vi "PDF_Interface_PDF Protokoll EPA1065_InterferenceVerification.vi"(8 "error in (no error)":errorcluster caption="Fehler (Eingang, kein Fehler)", 10 "Signalverlaufsdiagramm (Eingang)":refnum<vi>, 11 "Save PDF File Path":path) -> (0 "error out":errorcluster caption="Fehler (Ausgang)")   [LabVIEW 2020, in "EPA 1065.lvlib" / "HovaCAL Interference verificaton.lvlib"]
uses:
  HovaCAL Interference verificaton.lvlib
  Tabelle.ctl
  Tabelle Referenz.ctl
  Sprachverwaltung/FGV Aktion Tabelle zerlegen.ctl
  Aktion Index uebersetzten.ctl
  Aktion FGV Interference.ctl
  PDF_Interface/PDF Protokoll Standard Kopf Optionen.ctl
  <vilib>/Simplicity AI/SAI_PDF_API/Classes/Context/Controls/SAI_PDF_PDF Details.ctl
  PDF_Interface/PDF Interface Helper/PDFContentType.ctl
  PDF_Interface/PDF Interface Helper/PDFTableContentType.ctl
  PDF_Interface/PDF Interface Helper/PDFResults.ctl
  PDF_Interface/PDF Interface Helper/PDFResultPictures.ctl
  PDF_Interface/PDF Interface Helper/PDFCommentPosition.ctl
  PDF_Interface/PDF Interface Helper/PDFPageBreak.ctl
  PDF_Interface/PDF Interface Helper/PDFTablePictures.ctl
  PDF_Interface/PDF Interface Helper/PDFBemerkung.ctl
  <vilib>/Simplicity AI/SAI_PDF_API/Classes/Context/Controls/SAI_PDF_Text Align.ctl
  <vilib>/Simplicity AI/SAI_PDF_API/Classes/Context/Controls/SAI_PDF_Font.ctl
  <vilib>/Simplicity AI/SAI_PDF_API/Classes/Context/Controls/SAI_PDF_Font Encoding.ctl
  PDF_Interface/PDF Interface Helper/PDFGraph.ctl
  Sprachverwaltung/Sprachverwaltung.lvlib
  PDF_Interface/PDF Interface.lvlib
  PDF_Interface/PDF Interface Helper/PDF Interface Helper.lvlib
  <vilib>/Simplicity AI/SAI_PDF_API/Classes/Context/Context.lvclass
  Linearisierung V2/Protokoll/Protokoll.lvlib
panel:
  out "Kontroll Interferent":T1 caption="Kontroll-Interferent"
  out "Referenz Interferent":T2 caption="Referenz-Interferent"
  out "Komponente":T1
  out "Header Tabelle":string[][](table) caption="Tabelle"
  # "HovaCAL Interference Verification"
  # "Result"
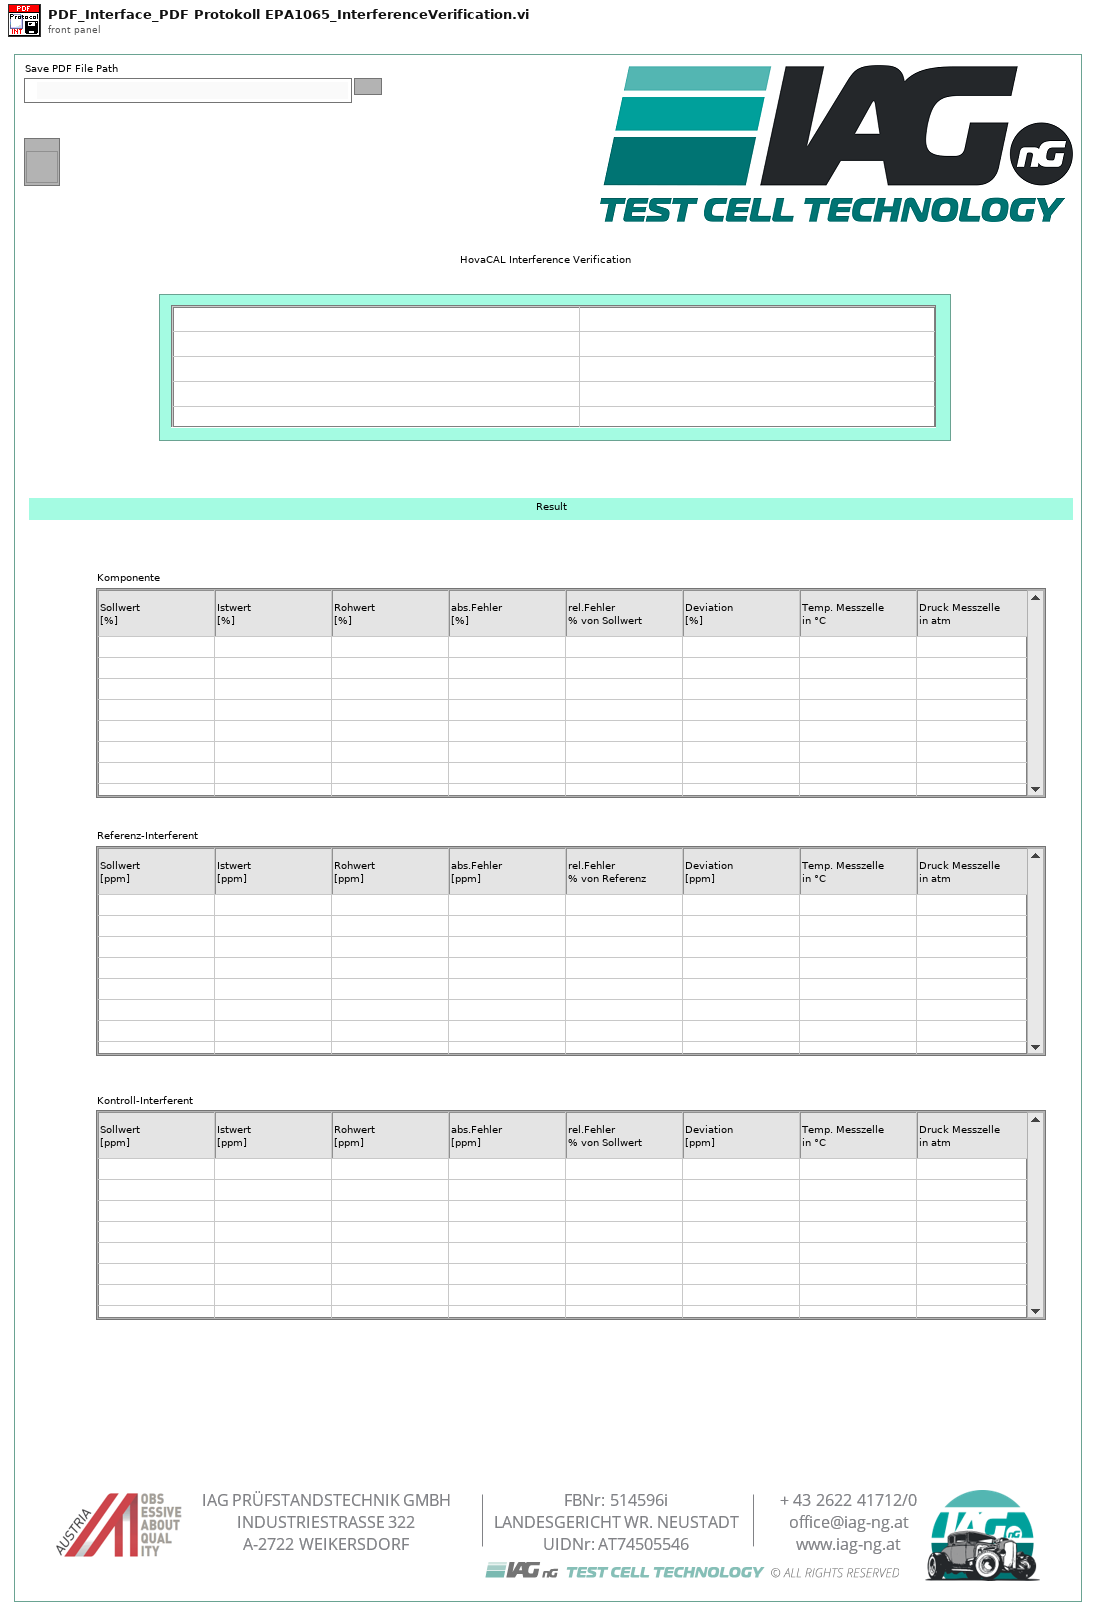
[diagram p1: front panel]
types:
  T1 = typedef "EPA 1065.lvlib/HovaCAL Interference verificaton.lvlib/Tabelle.ctl" = string[][]
  T2 = typedef "EPA 1065.lvlib/HovaCAL Interference verificaton.lvlib/Tabelle Referenz.ctl" = string[][]
  T3 = typedef "EPA 1065.lvlib/HovaCAL Interference verificaton.lvlib/Aktion FGV Interference.ctl" = enum16{"Lesen", "TestKonfig", "TestSetting", "Einheiten", "Ergebnis", "Laden", "Tabelle", "Speichern", "löschen"}
  T4 = typedef "EPA 1065.lvlib/HovaCAL Interference verificaton.lvlib/Aktion Index uebersetzten.ctl" = enum16{"lesen", "schreiben", "auswerten", "Referenzwert", "KompIndex", "RefInterferIndex", "KontrInterfIndex"}
  T5 = typedef "Sprachverwaltung.lvlib/FGV Aktion Tabelle zerlegen.ctl" = enum16{"laden", "vereinzeln", "speichern"}
  T6 = typedef "EPA 1065.lvlib/HovaCAL Interference verificaton.lvlib/Komponenten.ctl" = cluster{"Komponente":T7, "Komponente Index":i32, "Referenz Interferent":T7, "Refernz Interferent Index":i32, "Kontroll Interferent":T7, "Kontroll Interferent Index":i32, "Einheit Komponente":string, "Einheit Refernz Interferrent":string, "Einheit Kontroll Interferrent":string}
  T7 = typedef "String - Ausgabefeld.ctl" = string
  T8 = typedef "EPA 1065.lvlib/HovaCAL Interference verificaton.lvlib/TestSetting.ctl" = cluster{"Bearbeiter:":string, "Pfad:":path, "Textname:":string, "Analysator":T9}
  T9 = typedef "System Einstellungen V2.lvlib/Analysatoren.ctl" = string
  T10 = typedef "EPA 1065.lvlib/HovaCAL Interference verificaton.lvlib/TestKonfig.ctl" = cluster{"TestKonfig H2O":T11, "TestKonfig Interferent":T17}
  T11 = typedef "EPA 1065.lvlib/HovaCAL Interference verificaton.lvlib/TestKonfig H2O.ctl" = cluster{"Modus":T12, "Komponente:":u16, "Eingangs Konzentration:":dbl, "Einheit":T13, "Anzahl Stufen":sgl, "Zeitdauer Stufen":sgl, "Max Fehler":sgl, "zusätzliche Zeitdauer Erster Punkt":sgl, "Punkte umkehren":bool, "Stufen Tabelle":T14, "HovaCAL Flow Input Cluster":T15, "HovaCAL Temperature":T16}
  T12 = typedef "EPA 1065.lvlib/HovaCAL Interference verificaton.lvlib/Modus.ctl" = u16
  T13 = typedef "Linearisierung v2.lvlib/SpanEinstellungen.lvlib/Einheit.ctl" = enum16{"ppm", "%"}
  T14 = typedef "Linearisierung v2.lvlib/Gasteiler.lvlib/Stufen Tabelle 10 Stufen.ctl" = string[][]
  T15 = typedef "Linearisierung v2.lvlib/Gasteiler.lvlib/HovaCAL_Interface.lvlib/Controls.lvlib/Flow Einstellung.ctl" = cluster{"HovaCAL Flow Input Cluster":dbl}
  T16 = typedef "Linearisierung v2.lvlib/Gasteiler.lvlib/HovaCAL_Interface.lvlib/Controls.lvlib/Temp Sollwerte Anzeige.ctl" = dbl[]
  T17 = typedef "EPA 1065.lvlib/HovaCAL Interference verificaton.lvlib/TestKonfig Interferents.ctl" = cluster{"MFC1":enum16{"MFC 1"}, "Eingangs Konzentration MFC1":dbl, "Einheit MFC1 Eingang":T13, "Ausgangs Konzentration MFC1":dbl, "Einheit MFC1 Ausgang":T13, "MFC2":T18, "Referenz-Interferent:":u16, "Gasflaschen Nr MFC2":string, "Accuracy MFC2":string, "Eingangs Konzentration MFC2":dbl, "Einheit MFC2 Eingang":T13, "Ausgangs Konzentration MFC2":dbl, "Einheit MFC2 Ausgang":T13, "MFC3":T18, "Kontroll-Interferent:":u16, "Gasflaschen Nr MFC3":string, "Accuracy MFC3":string, "Eingangs Konzentration MFC3":dbl, "Einheit MFC3 Eingang":T13, "Ausgangs Konzentration MFC3":dbl, "Einheit MFC3 Ausgang":T13, "Gasflasche MFC2":T19, "Gasflasche MFC3":T19}
  T18 = typedef "EPA 1065.lvlib/HovaCAL Interference verificaton.lvlib/MFCAuswahl.ctl" = u16
  T19 = typedef "System Einstellungen V2.lvlib/Gasflasche Auswahl.ctl" = u16
  T20 = typedef "PDF Interface.lvlib/PDF Protokoll Standard Kopf Optionen.ctl" = cluster{"Analysator":bool, "FT-IR Rezept":bool, "Gasteiler":bool, "Gas Komponente":bool, "Gas Flasche":bool, "LIN Protokoll":bool, "Operator":bool}
  T21 = typedef "PDF Interface.lvlib/PDF Interface Helper.lvlib/PDFPageBreak.ctl" = enum16{"none", "before", "after", "after comment"}
  T22 = typedef "PDF Interface.lvlib/PDF Interface Helper.lvlib/PDFCommentPosition.ctl" = enum16{"before", "after"}
  T23 = typedef "PDF Interface.lvlib/PDF Interface Helper.lvlib/PDFGraph.ctl" = cluster{"GraphCtl Refnum":refnum<vi>, "Wrap Text (F:No)":bool, "Hide Grid (F:No)":bool, "Scale (100%)":sgl, "Align (Left)":T24, "PositionBemerkung":T22, "PageBreak":T21}
  T24 = typedef "SAI_PDF_Toolkit.lvlib/Context.lvclass/SAI_PDF_Text Align.ctl" = i32
  T25 = typedef "PDF Interface.lvlib/PDF Interface Helper.lvlib/PDFContentType.ctl" = cluster{"Titel":string, "Header Table":string[][], "Table Array":T26[], "Bemerkungen":T30[]}
  T26 = typedef "PDF Interface.lvlib/PDF Interface Helper.lvlib/PDFTableContentType.ctl" = cluster{"TableHeader":string[], "Table":string[][], "Relative Column Widths (%)":sgl[], "Results":T27, "PositionBemerkung":T22, "PageBreak":T21, "TablePictures":T29, "Horizontal Align":i32}
  T27 = typedef "PDF Interface.lvlib/PDF Interface Helper.lvlib/PDFResults.ctl" = cluster{"Results":cluster{"Result Text":string, "Result":bool}[], "ResultPictures":T28, "use Pictures":bool, "Image Scale (%)":sgl, "Autoscale? (T)":bool, "Horizontal Align":i32, "Position":i32}
  T28 = typedef "PDF Interface.lvlib/PDF Interface Helper.lvlib/PDFResultPictures.ctl" = cluster{"Yes Ctl Refnum":refnum<vi>, "No Ctl Refnum":refnum<vi>}
  T29 = typedef "PDF Interface.lvlib/PDF Interface Helper.lvlib/PDFTablePictures.ctl" = cluster{"Ctl Refnum In":refnum<vi>[], "RowOrColumn":enum16{"Row", "Column"}, "IndexToInsert":u16, "Image Scale (%)":sgl[], "Autoscale? (T)":bool[], "Horizontal Align":i32}
  T30 = typedef "PDF Interface.lvlib/PDF Interface Helper.lvlib/PDFBemerkung.ctl" = cluster{"Bemerkung Text":string, "Align (Left)":T24, "Add Line Feeds (F:No)":bool, "Font":T31}
  T31 = typedef "SAI_PDF_Toolkit.lvlib/Context.lvclass/SAI_PDF_Font.ctl" = cluster{"Font":string, "Size":i32, "Colour":u32, "Bold":bool, "Italic":bool, "Underline":bool, "Strikethrough":bool, "Font Encoding":T32}
  T32 = typedef "SAI_PDF_Toolkit.lvlib/Context.lvclass/SAI_PDF_Font Encoding.ctl" = enum16{"Cp1252, WinANSI", "IdentityH", "IdentityV", "Cp1250", "Cp1257", "MacRoman"}
  T33 = typedef "SAI_PDF_Toolkit.lvlib/Context.lvclass/SAI_PDF_PDF Details.ctl" = cluster{"Title":string, "Subject":string, "Keywords":string, "Author":string, "Creator":string}
  T34 = cluster{"Header Footer Text Cluster":cluster{"Header Text":string, "Footer Text":string, "Time":string, "Page Number":string}, "PDF Details":T33}
  T35 = cluster{"Header Size":i32, "Column Ratio left":sgl[]}
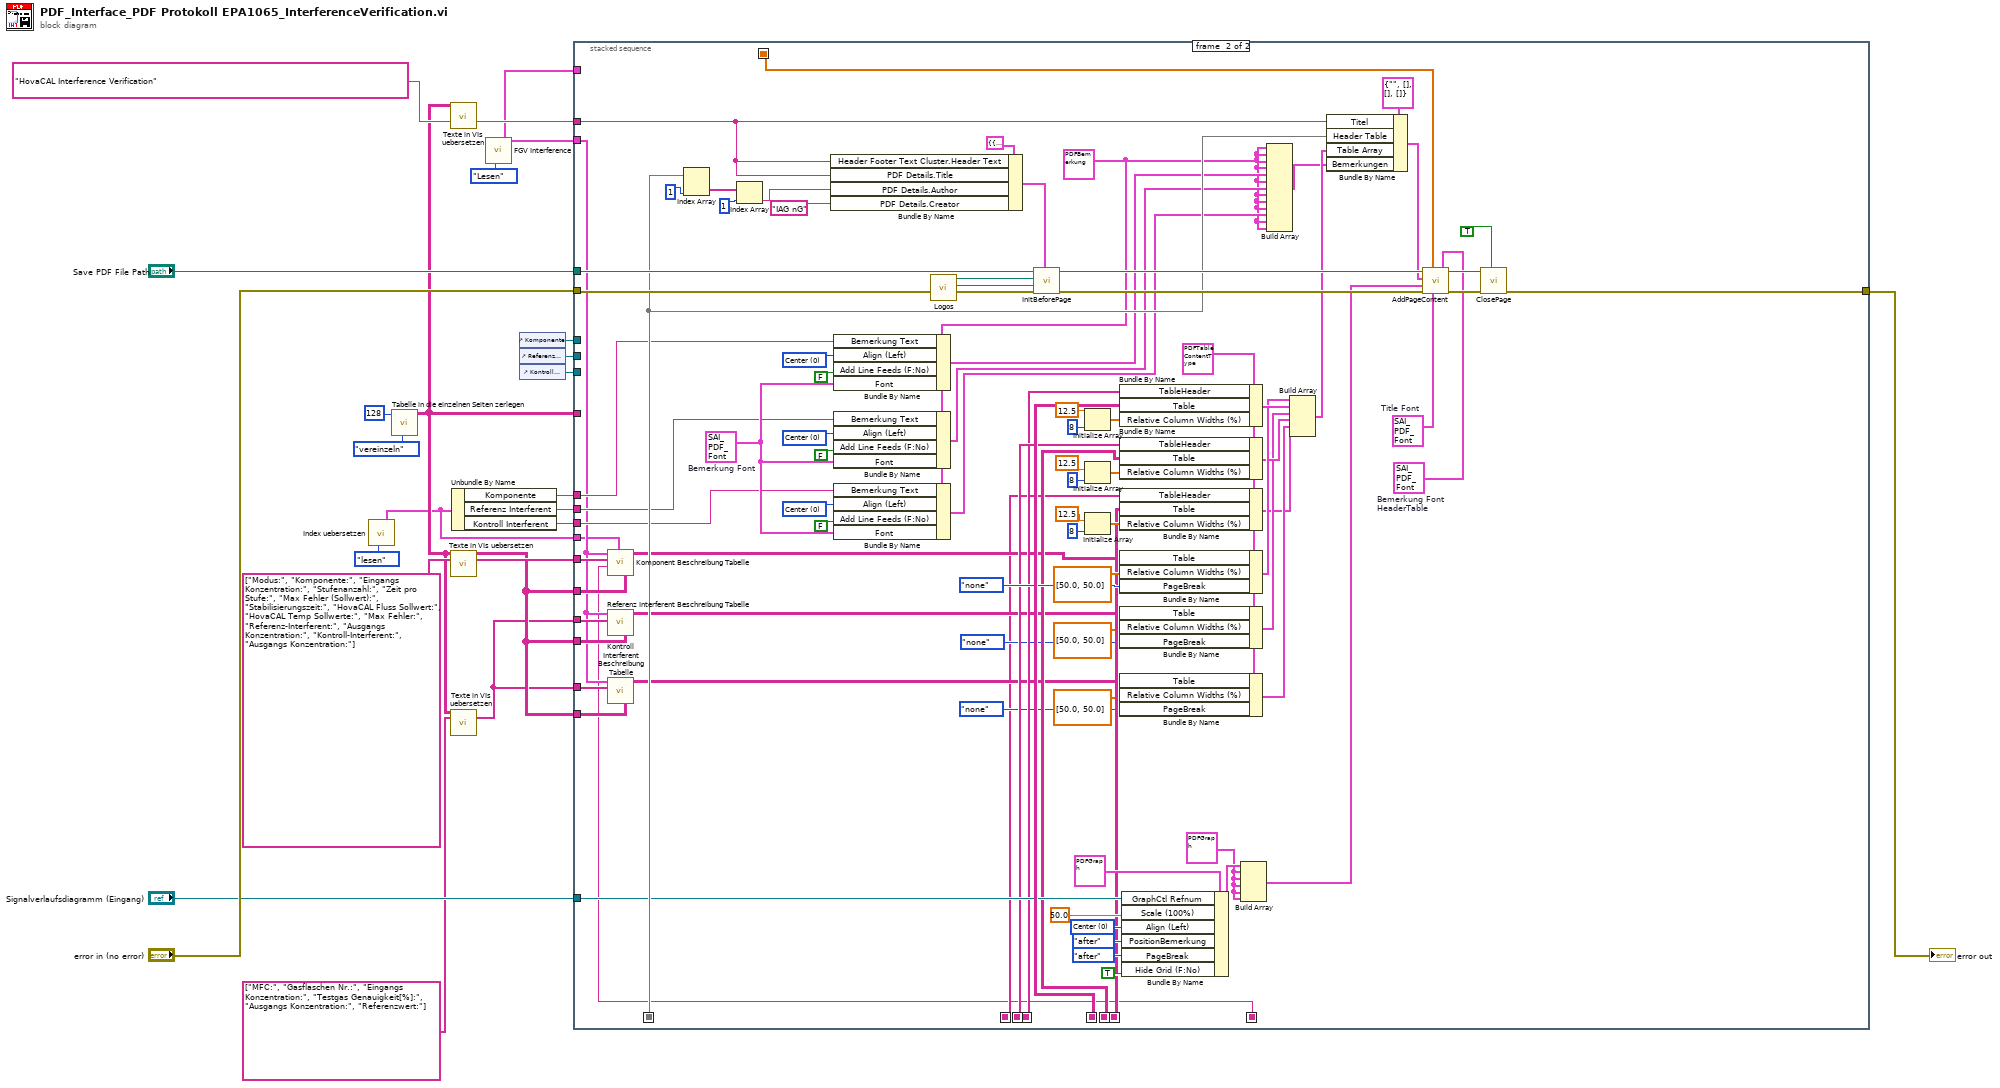
[diagram p0: block diagram]
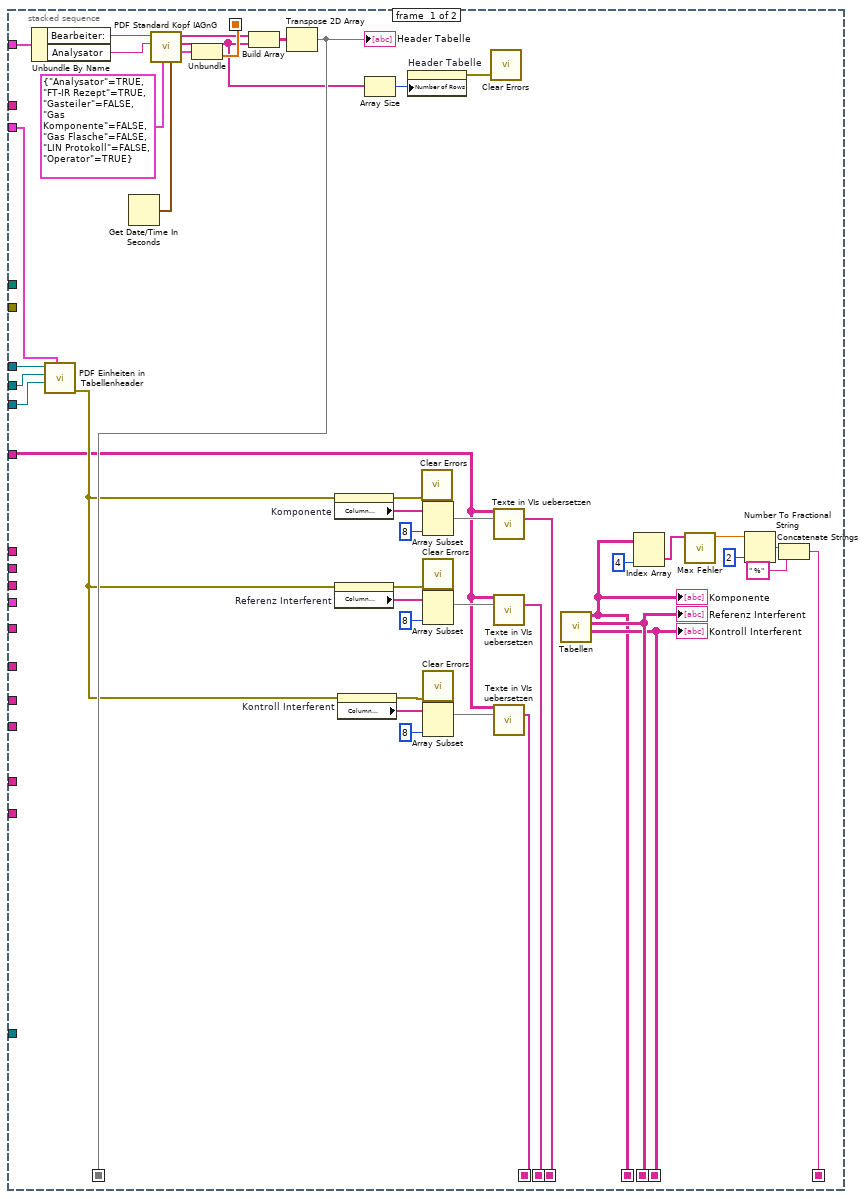
[diagram p2: hidden frame]
diagram:
  n1 = call "Index uebersetzen.vi"("Aktion"=Aktion_Index_uebersetzten."lesen") -> ("Komponenten"=w1:T6)  [unwired: 5 in, 5 out]
  n2 = call "Tabelle in die einzelnen Seiten zerlegen.vi"("Aktion"=FGV_Aktion_Tabelle_zerlegen."vereinzeln", "Index (Seite)"=128) -> ("Sprachliste"=w9:string[][])  [unwired: 7 in, 2 out]
  n3 = call "Texte in VIs uebersetzen.vi"("Sprachliste"=w9, "String zum Übersetzen"="HovaCAL Interference Verification") -> ("String zum Übersetzen"=w21:string)  [unwired: 9 in, 4 out]
  n4 = call "Texte in VIs uebersetzen.vi"("Sprachliste"=w9, "String-Array zum Übersetzen"=string[] ["Modus:", "Komponente:", "Eingangs Konzentration:", "Stufenanzahl:", "Zeit pro Stufe:", "Max Fehler (Sollwert):", "Stabilisierungszeit:", "HovaCAL Fluss Sollwert:", "HovaCAL Temp Sollwerte:", "Max Fehler:", "Referenz-Interferent:", "Ausgangs Konzentration:", "Kontroll-Interferent:", "Ausgangs Konzentration:"]) -> ("Sprachliste out"=w7:string[][], "String-Array zum Übersetzen"=w10:string[])  [unwired: 9 in, 3 out]
  n5 = call "Texte in VIs uebersetzen.vi"("Sprachliste"=w9, "String-Array zum Übersetzen"=string[] ["MFC:", "Gasflaschen Nr.:", "Eingangs Konzentration:", "Testgas Genauigkeit[%]:", "Ausgangs Konzentration:", "Referenzwert:"]) -> ("String-Array zum Übersetzen"=w6:string[])  [unwired: 9 in, 4 out]
  n6 = Unbundle By Name(w1) -> ("Komponente"=w17:T7, "Referenz Interferent"=w16:T7, "Kontroll Interferent"=w15:T7)
  n7 = call "FGV Interference.vi"("Aktion FGV Interference"=Aktion_FGV_Interference."Lesen") -> ("TestSetting"=w13:T8, "TestKonfig"=w12:T10)  [unwired: 9 in, 4 out]
  n8 = control-ref of="Komponente"() -> (w5:refnum<vi>)
  n9 = control-ref of="Referenz Interferent"() -> (w4:refnum<vi>)
  n10 = control-ref of="Kontroll Interferent"() -> (w3:refnum<vi>)
  n11 = stacked-sequence {
    seq-local: [w66 _] -> [_ w133]
    seq-local: [w33 _] -> [_ w139]
    seq-local: [w65 _] -> [_ w104]
    seq-local: [w55 _] -> [_ w124]
    seq-local: [w47 _] -> [_ w103]
    seq-local: [w46 _] -> [_ w102]
    seq-local: [w48 _] -> [_ w105]
    seq-local: [w34 _] -> [_ w72]
    seq-local: [w27 _] -> [_ w71]
    tunnel: w9 -> [w36 _]
    tunnel: "Save PDF File Path" -> [_ w142]
    tunnel: w21 -> [_ w143]
    tunnel: "error in (no error)" -> [_ w141]
    tunnel: [_ w140] -> w19
    tunnel: "Signalverlaufsdiagramm (Eingang)" -> [_ w117]
    tunnel: w17 -> [_ w100]
    tunnel: w16 -> [_ w99]
    tunnel: w15 -> [_ w98]
    tunnel: w13 -> [w45 _]
    tunnel: w12 -> [w41 w79]
    tunnel: w10 -> [_ w86]
    tunnel: w7 -> [_ w84]
    tunnel: w7 -> [_ w83]
    tunnel: w7 -> [_ w82]
    tunnel: w6 -> [_ w81]
    tunnel: w6 -> [_ w80]
    tunnel: w5 -> [w44 _]
    tunnel: w4 -> [w43 _]
    tunnel: w3 -> [w42 _]
    tunnel: w1 -> [_ w70]
    frame #0 {
      n12 = Unbundle By Name(w45) -> ("Bearbeiter:"=w59:string, "Analysator"=w58:T9)
      n13 = call "PDF Einheiten in Tabellenheader.vi"("TestKonfig"=w41, "Kontroll Interferent LIN Ausgabetabelle"=w42, "Referenz Interferent LIN Ausgabetabelle"=w43, "Tabelle (Eingang)"=w44) -> ("Fehler (Ausgang)"=w40:errorcluster)  [unwired: 7 in]
      n14 = Get Date/Time In Seconds() -> (seconds since 1Jan1904=w57:timestamp)
      n15 = call "PDF Standard Kopf IAGnG.vi"("Zeitstempel"=w57, "Oprtionen Cluster"=T20 {"Analysator"=TRUE, "FT-IR Rezept"=TRUE, "Gasteiler"=FALSE, "Gas Komponente"=FALSE, "Gas Flasche"=FALSE, "LIN Protokoll"=FALSE, "Operator"=TRUE}, "Analysator"=w58, "Bearbeiter/in"=w59) -> ("Size Cluster"=w56:T35, "Header Values"=w53:T7[], "Header Labels"=w54:string[])  [unwired: 4 in, 1 out]
      n16 = Unbundle(w56) -> ("Column Ratio left"=w55:sgl[])  [unwired: 1 out]
      n17 = Build Array(w54, w53) -> (w69:T7[][])
      n18 = Transpose 2D Array(2D array=w69) -> (transposed array=w66:T7[][])
      "Header Tabelle" <- w66
      n19 = property on="Komponente" class="Tbl (strikt)"(error in=w40) -> (error out=w62:errorcluster, "Column Headers[]"=w64:string[])  [unwired: 1 in, 1 out]
      n20 = property on="Referenz Interferent" class="Tbl (strikt)"(error in=w40) -> (error out=w52:errorcluster, "Column Headers[]"=w50:string[])  [unwired: 1 in, 1 out]
      n21 = property on="Kontroll Interferent" class="Tbl (strikt)"(error in=w40) -> (error out=w38:errorcluster, "Column Headers[]"=w37:string[])  [unwired: 1 in, 1 out]
      n22 = Array Size(array=w53) -> (size(s)=w68:i32)
      n23 = property on="Header Tabelle" class="Tbl (strikt)"("Number of Rows"=w68) -> (error out=w67:errorcluster)  [unwired: 2 in, 1 out]
      n24 = call <vilib>:"Clear Errors.vi"("error in (no error)"=w62) -> ()  [unwired: 5 in, 2 out]
      n25 = Array Subset(array=w64, length=8 ("Länge")) -> (w63:string[])  [unwired: 1 in]
      n26 = call <vilib>:"Clear Errors.vi"("error in (no error)"=w52) -> ()  [unwired: 5 in, 2 out]
      n27 = Array Subset(array=w50, length=8 ("Länge")) -> (w49:string[])  [unwired: 1 in]
      n28 = call <vilib>:"Clear Errors.vi"("error in (no error)"=w38) -> ()  [unwired: 5 in, 2 out]
      n29 = Array Subset(array=w37, length=8 ("Länge")) -> (w35:string[])  [unwired: 1 in]
      n30 = call <vilib>:"Clear Errors.vi"("error in (no error)"=w67) -> ()  [unwired: 5 in, 2 out]
      n31 = call "Texte in VIs uebersetzen.vi"("Sprachliste"=w36, "String-Array zum Übersetzen"=w63) -> ("String-Array zum Übersetzen"=w65:string[])  [unwired: 9 in, 4 out]
      n32 = call "Texte in VIs uebersetzen.vi"("Sprachliste"=w36, "String-Array zum Übersetzen"=w49) -> ("String-Array zum Übersetzen"=w48:string[])  [unwired: 9 in, 4 out]
      n33 = call "Texte in VIs uebersetzen.vi"("Sprachliste"=w36, "String-Array zum Übersetzen"=w35) -> ("String-Array zum Übersetzen"=w34:string[])  [unwired: 9 in, 4 out]
      n34 = call "Tabellen.vi"() -> ("Tabelle Kontroll Interferent"=w46:string[][], "Tabbelle Referenz Interferent"=w47:string[][], "Tabelle Komponente"=w33:string[][])  [unwired: 5 in, 4 out]
      "Komponente" <- w33
      "Referenz Interferent" <- w47
      "Kontroll Interferent" <- w46
      n35 = Index Array(array=w33, index (col)=4 ("Deaktivierter Index (Spalte)")) -> (element=w29:string[])  [unwired: 1 in]
      n36 = call "Max Fehler.vi"("Tabelle"=w29) -> ("max Fehler"=w28:dbl)  [unwired: 10 in]
      n37 = Number To Fractional String(number=w28, precision (6)=i16 2 ("Genauigkeit (6)")) -> (F-format string=w30:string)  [unwired: 2 in]
      n38 = Concatenate Strings(w30, " %" ("String")) -> (w27:string)
    }
    frame #1 {
      w119 = T24 0 items=["Center", "Justified", "Justified All", "Left", "Right"] ("Align (Left)")
      w87 = T23 {"GraphCtl Refnum"=refnum, "Wrap Text (F:No)"=FALSE, "Hide Grid (F:No)"=FALSE, "Scale (100%)"=0.0, "Align (Left)"=0, "PositionBemerkung"=enum."before", "PageBreak"=enum."after comment"} ("Element")
      w126 = T31 {"Font"="Arial", "Size"=12, "Colour"=0, "Bold"=TRUE, "Italic"=TRUE, "Underline"=FALSE, "Strikethrough"=FALSE, "Font Encoding"=enum."Cp1252, WinANSI"}  # Bemerkung Font
      w73 = T30 {"Bemerkung Text"="", "Align (Left)"=0, "Add Line Feeds (F:No)"=FALSE, "Font"={"Font"="Arial", "Size"=10, "Colour"=0, "Bold"=FALSE, "Italic"=FALSE, "Underline"=FALSE, "Strikethrough"=FALSE, "Font Encoding"=enum."Cp1252, WinANSI"}} ("Bemerkung")
      w91 = T26 {"TableHeader"=[], "Table"=[], "Relative Column Widths (%)"=[], "Results"={"Results"=[], "ResultPictures"={"Yes Ctl Refnum"=refnum, "No Ctl Refnum"=refnum}, "use Pictures"=FALSE, "Image Scale (%)"=0.0, "Autoscale? (T)"=FALSE, "Horizontal Align"=0, "Position"=0}, "PositionBemerkung"=enum."before", "PageBreak"=enum."none", "TablePictures"={"Ctl Refnum In"=[], "RowOrColumn"=enum."Row", "IndexToInsert"=0, "Image Scale (%)"=[], "Autoscale? (T)"=[], "Horizontal Align"=0}, "Horizontal Align"=0} ("Table Array")
      w128 = T24 0 items=["Center", "Justified", "Justified All", "Left", "Right"] ("Align (Left)")
      w134 = T24 0 items=["Center", "Justified", "Justified All", "Left", "Right"] ("Align (Left)")
      w137 = T24 0 items=["Center", "Justified", "Justified All", "Left", "Right"] ("Align (Left)")
      w74 = T31 {"Font"="Arial", "Size"=10, "Colour"=16777222, "Bold"=FALSE, "Italic"=FALSE, "Underline"=FALSE, "Strikethrough"=FALSE, "Font Encoding"=enum."Cp1252, WinANSI"}  # Bemerkung Font HeaderTable
      w146 = T31 {"Font"="Arial", "Size"=24, "Colour"=0, "Bold"=TRUE, "Italic"=FALSE, "Underline"=TRUE, "Strikethrough"=FALSE, "Font Encoding"=enum."Cp1252, WinANSI"}  # Title Font
      n39 = call "Komponent Beschreibung Tabelle.vi"("Sprachliste"=w84, "Komponenten"=w70, "Max Fehler"=w71, "Table Header"=w86, "TestKonfig"=w79) -> ("Tabelle"=w85:string[][])  [unwired: 6 in]
      n40 = call "Referenz Interferent Beschreibung Tabelle.vi"("Sprachliste"=w83, "Table Header"=w81, "TestKonfig"=w79) -> ("Tabelle"=w78:string[][])  [unwired: 8 in]
      n41 = call "Kontroll Interferent Beschreibung Tabelle.vi"("Sprachliste"=w82, "Table Header"=w80, "TestKonfig"=w79) -> ("Tabelle"=w77:string[][])  [unwired: 8 in]
      n42 = Index Array(array=w133, index (col)=1 ("Index")) -> (element=w131:T7[])  [unwired: 1 in]
      n43 = Index Array(array=w131, index=1 ("Index")) -> (element=w144:T7)
      n44 = Bundle By Name(cluster=T34 {"Header Footer Text Cluster"={"Header Text"="Protokoll XYZ", "Footer Text"="IAG nG", "Time"="<TIMESTAMP yyyy-MM-dd>", "Page Number"="Page <P> of <PT>"}, "PDF Details"={"Title"="Test PDF", "Subject"="Versa Tabasco", "Keywords"="", "Author"="RIW", "Creator"="IAG"}} ("Info"), "Header Footer Text Cluster.Header Text"=w143, "PDF Details.Title"=w143, "PDF Details.Author"=w144, "PDF Details.Creator"="IAG nG") -> (w150:T34)
      n45 = Bundle By Name(cluster=w73, "Bemerkung Text"=w100, "Align (Left)"=w128, "Add Line Feeds (F:No)"=FALSE, "Font"=w126) -> (w127:T30)
      n46 = Bundle By Name(cluster=w73, "Bemerkung Text"=w99, "Align (Left)"=w137, "Add Line Feeds (F:No)"=FALSE, "Font"=w126) -> (w76:T30)
      n47 = Bundle By Name(cluster=w73, "Bemerkung Text"=w98, "Align (Left)"=w134, "Add Line Feeds (F:No)"=FALSE, "Font"=w126) -> (w75:T30)
      n48 = call "Logos.vi"() -> ("Footer Image File Path"=w158:path, "Header Image File Path"=w159:path)  [unwired: 8 in, 2 out]
      n49 = call "InitBeforePage.vi"("Info"=w150, "Fehler (Eingang, kein Fehler)"=w141, "Footer Image File Path"=w158, "Header Image File Path"=w159, "Path (Dialog if Empty)"=w142) -> ("Fehler (Ausgang)"=w157:errorcluster, "Context (Ausgang)"=w156:refnum<class "Context.lvclass">)  [unwired: 5 in]
      n50 = Initialize Array(12.5 ("Element"), 8 ("Dimensionsgröße")) -> (w113:dbl[])
      n51 = Initialize Array(12.5 ("Element"), 8 ("Dimensionsgröße")) -> (w108:dbl[])
      n52 = Initialize Array(12.5 ("Element"), 8 ("Dimensionsgröße")) -> (w109:dbl[])
      n53 = Bundle By Name(cluster=w91, "TableHeader"=w104, "Table"=w139, "Relative Column Widths (%)"=w113) -> (w111:T26)
      n54 = Bundle By Name(cluster=w91, "TableHeader"=w105, "Table"=w103, "Relative Column Widths (%)"=w108) -> (w92:T26)
      n55 = Bundle By Name(cluster=w91, "TableHeader"=w72, "Table"=w102, "Relative Column Widths (%)"=w109) -> (w88:T26)
      n56 = Bundle By Name(cluster=w91, "Table"=w85, "Relative Column Widths (%)"=sgl[] [50.0, 50.0], "PageBreak"=PDFPageBreak."none") -> (w95:T26)
      n57 = Bundle By Name(cluster=w91, "Table"=w78, "Relative Column Widths (%)"=sgl[] [50.0, 50.0], "PageBreak"=PDFPageBreak."none") -> (w90:T26)
      n58 = Bundle By Name(cluster=w91, "Table"=w77, "Relative Column Widths (%)"=sgl[] [50.0, 50.0], "PageBreak"=PDFPageBreak."none") -> (w89:T26)
      n59 = Bundle By Name(cluster=T23 {"GraphCtl Refnum"=refnum, "Wrap Text (F:No)"=FALSE, "Hide Grid (F:No)"=FALSE, "Scale (100%)"=100.0, "Align (Left)"=0, "PositionBemerkung"=enum."before", "PageBreak"=enum."after comment"} ("Graph"), "GraphCtl Refnum"=w117, "Scale (100%)"=sgl 50.0, "Align (Left)"=w119, "PositionBemerkung"=PDFCommentPosition."after", "PageBreak"=PDFPageBreak."after", "Hide Grid (F:No)"=TRUE) -> (w116:T23)
      n60 = Build Array(w116, w87, w87, w87, w87, w87) -> (w101:T23[])
      n61 = Build Array(w73, w73, w73, w73, w127, w73, w76, w73, w73, w73, w75, w73, w73) -> (w138:T30[])
      n62 = Build Array(w95, w111, w90, w92, w89, w88) -> (w148:T26[])
      n63 = Bundle By Name(cluster=T25 {"Titel"="", "Header Table"=[], "Table Array"=[], "Bemerkungen"=[]} ("Content"), "Titel"=w143, "Header Table"=w133, "Table Array"=w148, "Bemerkungen"=w138) -> (w147:T25)
      n64 = call "AddPageContent.vi"("HeaderTableFont"=w74, "Title Font"=w146, "Column Ratio left"=w124, "error in"=w157, "Graph Array"=w101, "Content"=w147, "Context (Eingang)"=w156) -> ("error out"=w155:errorcluster, "Context (Ausgang)"=w154:refnum<class "Context.lvclass">)  [unwired: 3 in]
      n65 = call "ClosePage.vi"("popup viewer"=TRUE, "Fehler (Eingang, kein Fehler)"=w155, "Context (Eingang)"=w154) -> ("Fehler (Ausgang)"=w140:errorcluster)  [unwired: 8 in]
    }
  }
  "error out" <- w19
